vi "acelerador.vi"() -> ()   [LabVIEW 2011]
panel:
  in  "Boolean":bool
  in  "OK Button 2":bool
  in  "OK Button":bool
  out "Velocidad":i32(knob) scale=0.0..220.0
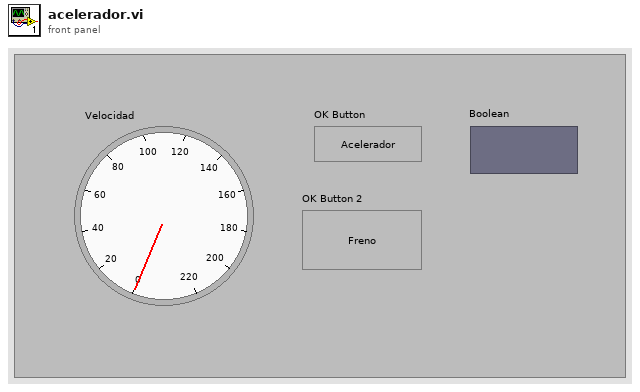
[diagram p1: front panel]
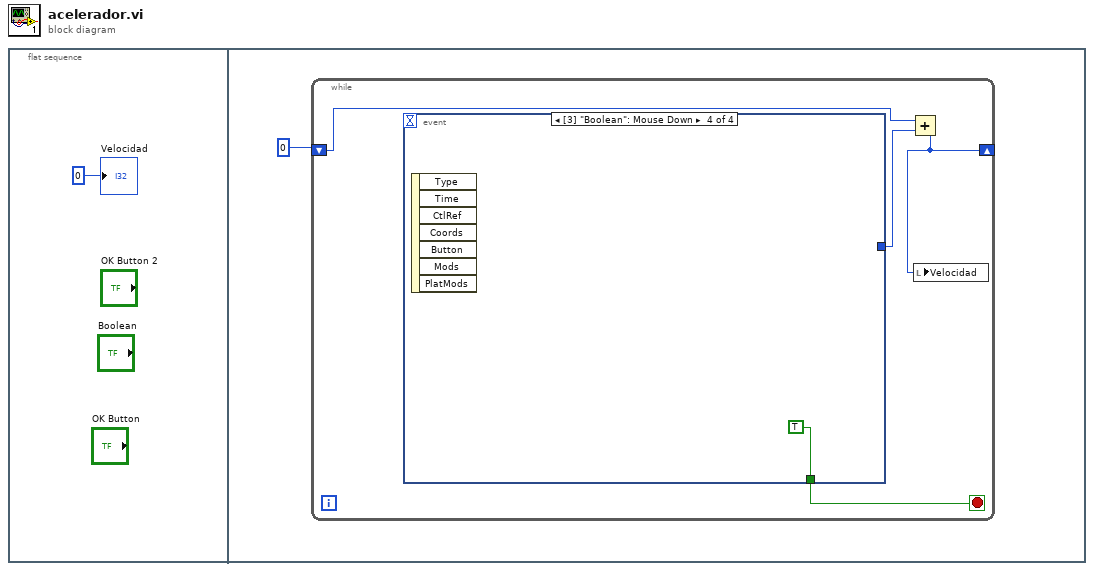
[diagram p0: block diagram]
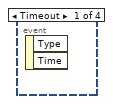
[diagram p2: hidden frame]
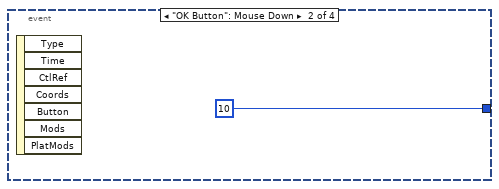
[diagram p3: hidden frame]
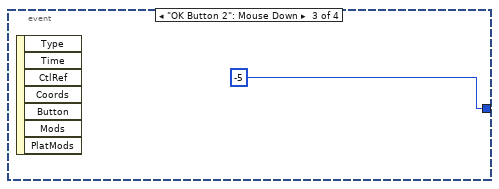
[diagram p4: hidden frame]
diagram:
  n1 = flat-sequence {
    frame #0 {
      "Velocidad" <- 0
    }
    frame #1 {
      n2 = while {
        shift-right: [w4] -> _
        shift-left: 0 -> [w6]
        stop <- w3 stop-if-true
        n3 = event shown="[3] \"Boolean\": Mouse Down" {
          selector: _ -> [_ _ _ _]
          dyn-events: _ -> [_ _ _ _]
          timeout: _ -> [_ _ _ _]
          tunnel: [_ 10 -5 _] -> w5
          tunnel: [_ _ _ TRUE] -> w3
          event Timeout {
            n4 = event-data() -> ()  [unwired: 1 in, 2 out]
          }
          event "OK Button": Mouse Down {
            n5 = event-data() -> ()  [unwired: 1 in, 7 out]
          }
          event "OK Button 2": Mouse Down {
            n6 = event-data() -> ()  [unwired: 1 in, 7 out]
          }
          event "Boolean": Mouse Down {
            n7 = event-data() -> ()  [unwired: 1 in, 7 out]
          }
        }
        n8 = Add(x=w6, y=w5) -> (x+y=w4:i32)
        n9 = local write "Velocidad"(w4) -> ()
      }
    }
  }
